vi "报表查询.vi"(11 "ConnectString":string="\"Provider=Microsoft.Jet.OLEDB.4.0;Data Source=C:\\\\Users\\\\Public\\\\Documents\\\\National \n\nInstruments\\\\TestStand 2017 (32-bit)\\\\Components\\\\Models\\\\TestStand Results.mdb;Persist Security Info=False\"") -> ()   [LabVIEW 2018, in "TestStand Simple UI.lvlib"]
uses:
  TestExec.llb/TestStand Simple UI.lvlib
  <vilib>/addons/database/Connection.llb/Conn ObjectReference.ctl
  <vilib>/addons/database/Connection.llb/DB Tools Open Connec (String).vi
  <vilib>/addons/database/Connection.llb/Conn Execute.vi
  <vilib>/addons/database/Recordset.llb/Rec Fetch Recordset Data (R).vi
  <vilib>/addons/database/Recordset.llb/Rec Destroy - Connection.vi
  <vilib>/Utility/file.llb/Write Delimited Spreadsheet (string).vi
  <vilib>/addons/database/_DB Variant To Data/Database Variant To Data.xnode
  <vilib>/addons/database/NI_Database_API.lvlib
panel:
  out "connection reference":T1
  out "error out":errorcluster
  in  "预览":bool
  in  "保存按钮":bool
  in  "搜索按钮":bool
  in  "二维码":string
  out "SN":string
  out "Row":i32
  in  "筛选结果":i32(listbox)
  in  "步骤结果":i32(listbox)
  in  "关键步骤":i32(listbox)
  out "data 2":string[][](array[string])
  out "tables":string[](array[string])
  in  "预览数据":i32(listbox)
  out "data 6":string[][](array[string])
  out "data 5":string[][](array[string])
  out "data 4":string[][](array[string])
  out "data 3":string[][](array[string])
  in  "测试报表":i32(listbox)
  out "data":string[][](array[string])
  in  "树形":string(tree)
  # "测试报表查询"
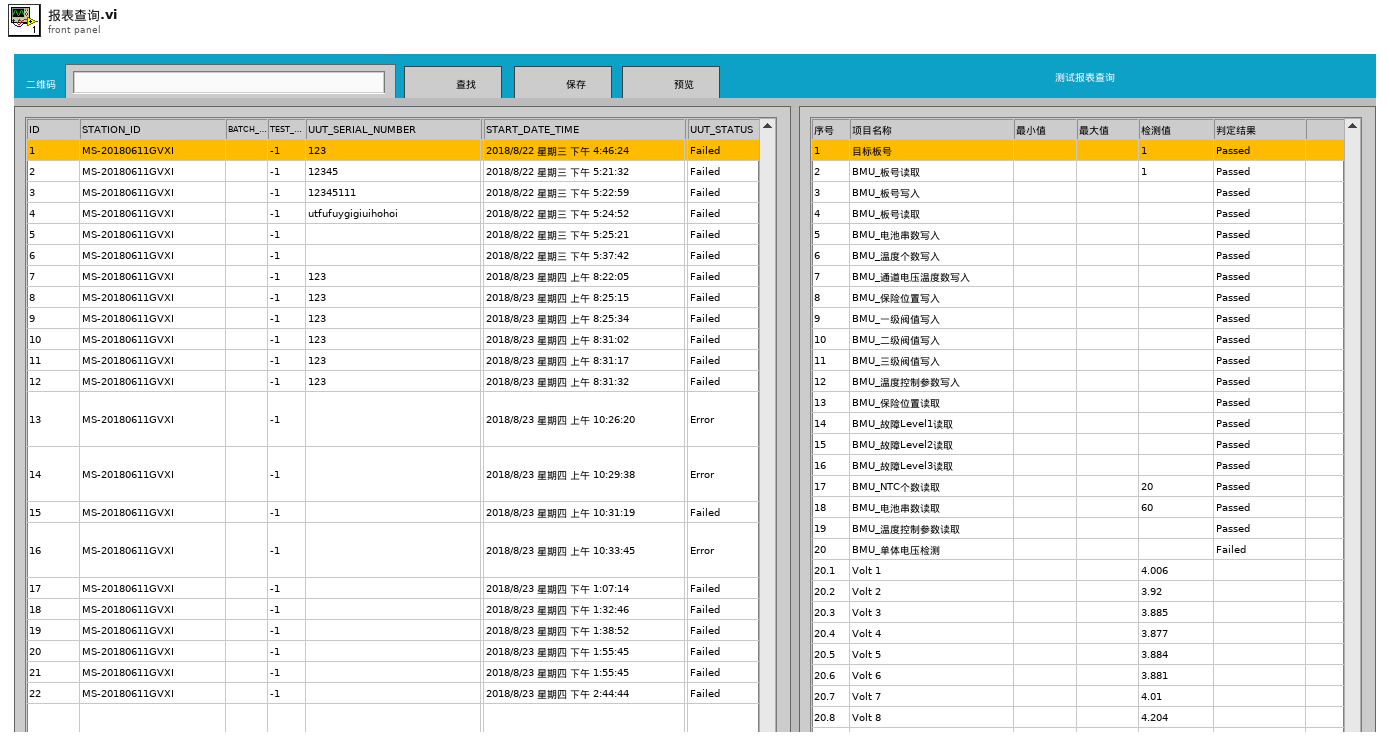
[diagram p1: front panel]
types:
  T1 = typedef "NI_Database_API.lvlib/Conn ObjectReference.ctl" = refnum<k1>
  T2 = typedef "LVPoint32TypeDef.ctl" = cluster{"Horizontal":i32, "Vertical":i32}
  T3 = typedef "LVRowAndColumnTypeDef.ctl" = cluster{"Row":i32, "Column":i32}
  T4 = typedef "NI_Database_API.lvlib/Rec ObjectReference.ctl" = refnum<k1>
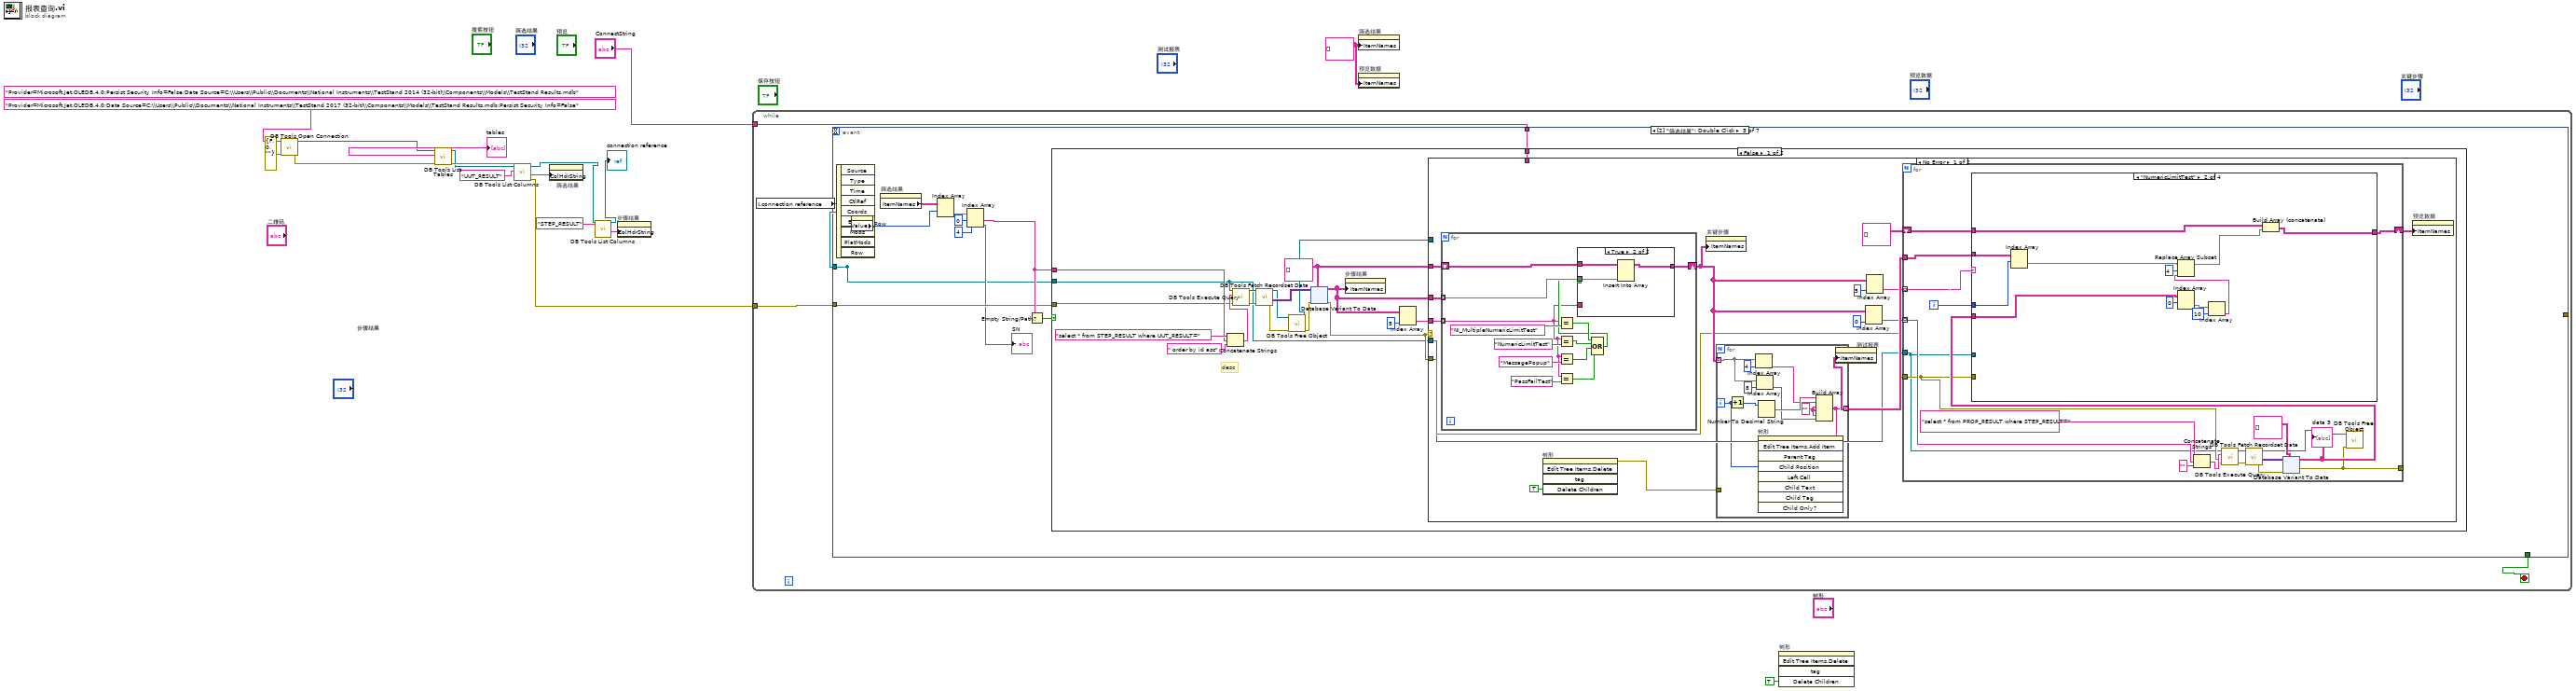
[diagram p0: block diagram]
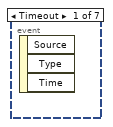
[diagram p2: hidden frame]
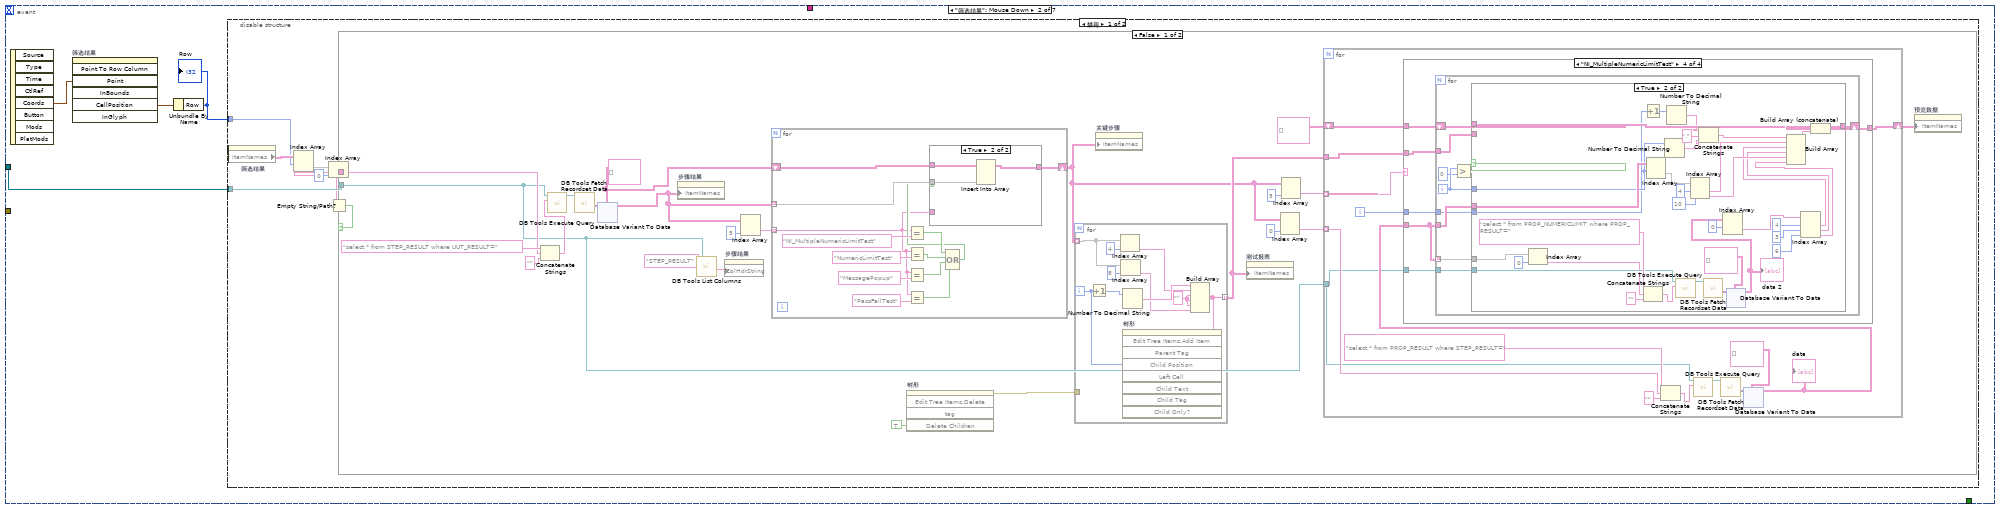
[diagram p3: hidden frame]
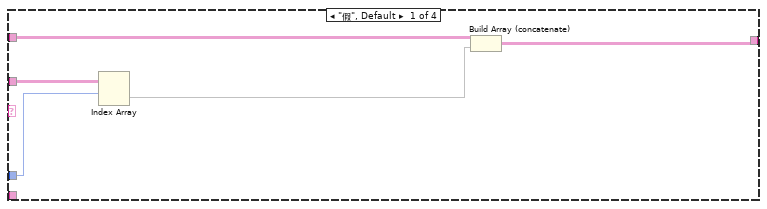
[diagram p4: hidden frame]
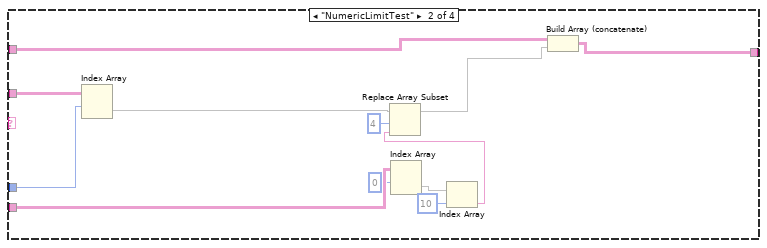
[diagram p5: hidden frame]
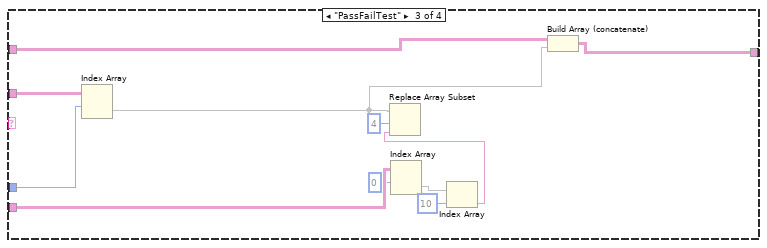
[diagram p6: hidden frame]
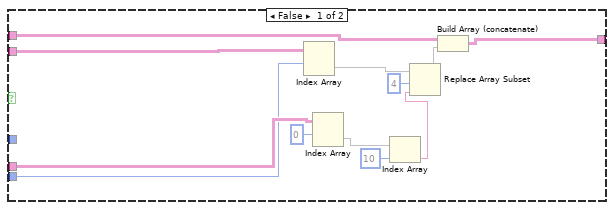
[diagram p7: hidden frame]
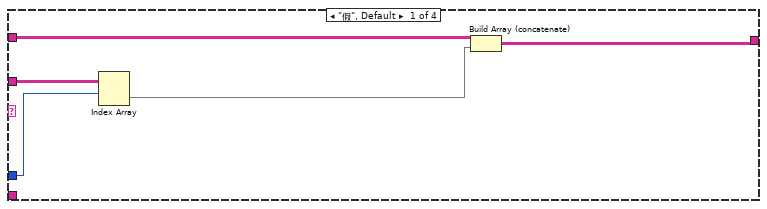
[diagram p11: hidden frame]
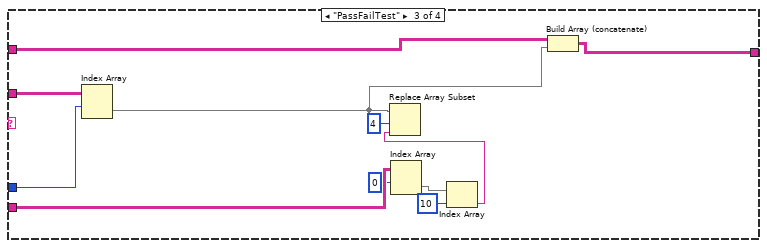
[diagram p12: hidden frame]
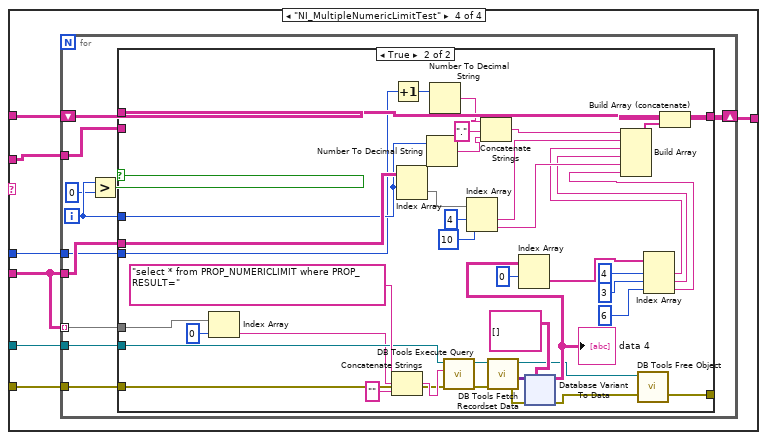
[diagram p13: hidden frame]
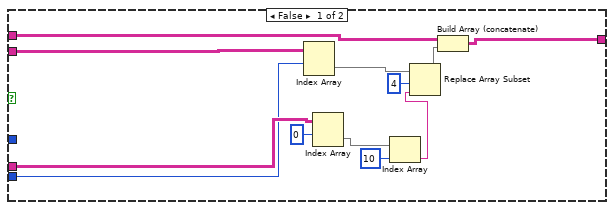
[diagram p14: hidden frame]
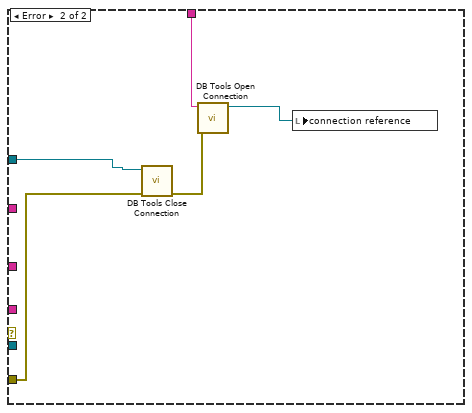
[diagram p16: hidden frame]
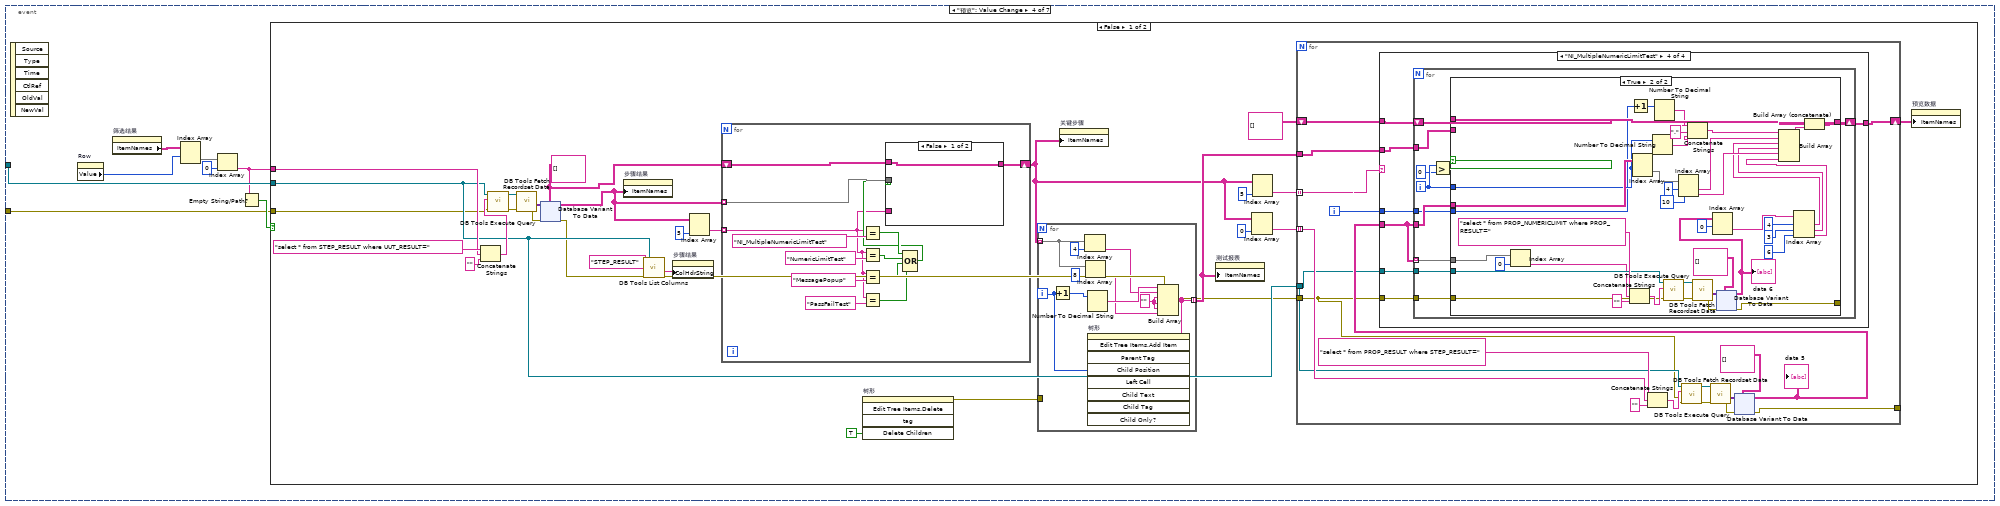
[diagram p18: hidden frame]
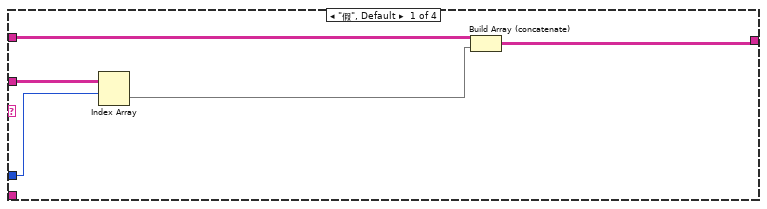
[diagram p19: hidden frame]
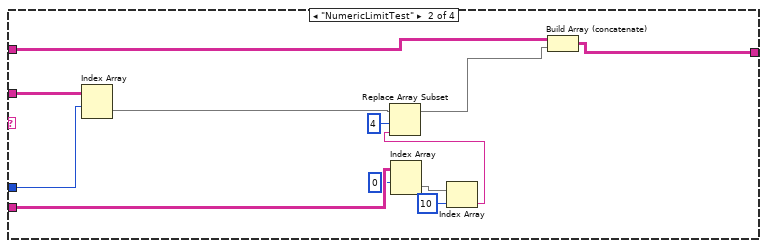
[diagram p20: hidden frame]
diagram:
  w2 = string[][] [] ("Item Names")
  (unwired) "Provider=Microsoft.Jet.OLEDB.4.0;Persist Security Info=False;Data Source=C:\\Users\\Public\\Documents\\National Instruments\\TestStand 2014 (32-bit)\\Components\\Models\\TestStand Results.mdb"
  n1 = call-poly <vilib>:"DB Tools Open Connection.vi"("error in (no error)"=errorcluster {"status"=FALSE, "code"=0, "source"=""}, "connection information"="Provider=Microsoft.Jet.OLEDB.4.0;Data Source=C:\\Users\\Public\\Documents\\National Instruments\\TestStand 2017 (32-bit)\\Components\\Models\\TestStand Results.mdb;Persist Security Info=False") -> ("error out"=w11:errorcluster, "connection reference"=w14:T1)  [unwired: 6 in]
  n2 = call <vilib>:"DB Tools List Tables.vi"("error in (no error)"=w11, "connection reference"=w14) -> ("error out"=w10:errorcluster, "tables"=→"tables":string[], "connection reference out"=w8:T1)  [unwired: 3 in]
  n3 = call <vilib>:"DB Tools List Columns.vi"("error in (no error)"=w10, "table"="UUT_RESULT", "connection reference"=w8) -> ("error out"=w9:errorcluster, "columns"=w15:string[], "connection reference out"=w5:T1)  [unwired: 1 in, 1 out]
  n4 = property on="筛选结果" class="MCListbox (strict)"("ColHdrString"=w15) -> ()  [unwired: 2 in, 2 out]
  n5 = call <vilib>:"DB Tools List Columns.vi"("table"="STEP_RESULT", "connection reference"=w5) -> ("columns"=w7:string[], "connection reference out"=→"connection reference":T1)  [unwired: 2 in, 2 out]
  n6 = property on="步骤结果" class="MCListbox (strict)"("ColHdrString"=w7) -> ()  [unwired: 2 in, 2 out]
  n7 = while {
    tunnel: w9 -> [w21]
    tunnel: "ConnectString" -> [w19]
    stop <- w20 stop-if-true
    n8 = local read "connection reference"() -> (w18:T1)
    n9 = event shown="[2] \"筛选结果\": Double Click" {
      selector: _ -> [_ _ _ _ _ _ _]
      dyn-events: _ -> [_ _ _ _ _ _ _]
      timeout: _ -> [_ _ _ _ _ _ _]
      tunnel: w18 -> [_ w23 w320 w650 _ w969 w974]
      tunnel: w21 -> [_ _ w324 w646 _ w968 w972]
      tunnel: [_ _ _ _ _ w970 _] -> w20
      tunnel: [_ _ _ _ _ _ w971] -> _
      tunnel: w19 -> [_ _ w321 _ _ _ _]
      tunnel: [_ _ w320 _ _ _ _] -> _
      event Timeout {
        n10 = event-data() -> ()  [unwired: 1 in, 3 out]
      }
      event "筛选结果": Mouse Down {
        n11 = event-data() -> ("Coords"=w25:T2)  [unwired: 1 in, 7 out]
        n12 = invoke on="筛选结果" class="MCListbox (严格)" method="Point To Row Column"("Point"=w25) -> ("CellPosition"=w24:T3)  [unwired: 6 in, 6 out]
        n13 = Unbundle By Name(w24) -> ("Row"=w22:i32)
        "Row" <- w22
        n14 = disable-structure shown="禁用" {
          disable-tunnel: w23 -> [w29 _]
          disable-tunnel: w22 -> [w28 _]
          frame Disabled {
            n15 = property on="筛选结果" class="MCListbox (strict)"() -> ("ItemNames"=w32:string[][])  [unwired: 2 in, 2 out]
            n16 = Index Array(array=w32, index (row)=w28) -> (element=w31:string[])  [unwired: 1 in]
            n17 = Index Array(array=w31, index=0 ("索引")) -> (element=w27:string)
            n18 = Empty String/Path?(string/path=w27) -> (empty?=w26:bool)
            n19 = case shown="False" w26 {
              tunnel: w29 -> [w37 _]
              tunnel: w27 -> [w49 _]
              frame False {
                w44 = string[][] []
                n20 = Concatenate Strings("select * from STEP_RESULT where UUT_RESULT=" ("condition"), w49, "" ("字符串")) -> (w51:string)
                n21 = call-poly <vilib>:"DB Tools Execute Query.vi"("SQL query"=w51, "connection reference"=w37) -> ("recordset reference"=w55:T4)  [unwired: 6 in, 1 out]
                n22 = call-poly <vilib>:"DB Tools Fetch Recordset Data.vi"("recordset reference"=w55) -> ("recordset data"=w54:variant[][])  [unwired: 4 in, 2 out]
                n23 = xnode "Database Variant To Data"("database variant"=w54, "type"=w44) -> ("data"=w45:string[][])  [unwired: 1 in, 1 out]
                n24 = property on="步骤结果" class="MCListbox (strict)"("ItemNames"=w45) -> ()  [unwired: 2 in, 2 out]
                n25 = call <vilib>:"DB Tools List Columns.vi"("table"="STEP_RESULT", "connection reference"=w37) -> ("columns"=w48:string[])  [unwired: 2 in, 3 out]
                n26 = property on="步骤结果" class="MCListbox (strict)"("ColHdrString"=w48) -> ()  [unwired: 2 in, 2 out]
                n27 = Index Array(array=w45, index (col)=5 ("禁用的索引 (列)")) -> (element=w46:string[])  [unwired: 1 in]
                n28 = for {
                  tunnel: w46 -> [w260] mode=indexing
                  tunnel: w45 -> [w264] mode=indexing
                  shift-right: [w262] -> w39
                  shift-left: w44 -> [w265]
                  n29 = Equal?(x=w260, y="NI_MultipleNumericLimitTest") -> (x = y?=w268:bool)
                  n30 = Equal?(x=w260, y="NumericLimitTest") -> (x = y?=w267:bool)
                  n31 = Equal?(x=w260, y="MessagePopup") -> (x = y?=w266:bool)
                  n32 = Equal?(x=w260, y="PassFailTest") -> (x = y?=w259:bool)
                  n33 = Compound Arithmetic op=OR(w268, w267, w266, w259) -> (w263:bool)
                  n34 = case shown="True" w263 {
                    tunnel: w265 -> [w272 w275]
                    tunnel: w264 -> [_ w274]
                    tunnel: [w272 w273] -> w262
                    tunnel: w260 -> [_ _]
                    frame False {
                    }
                    frame True {
                      n35 = Insert Into Array(array=w275, new element=w274) -> (w273:string[][])  [unwired: 2 in]
                    }
                  }
                }
                n36 = invoke on="树形" class="Tree (严格)" method="Edit Tree Items.Delete"("Delete Children"=TRUE ("删除子项？")) -> (error out=w35:errorcluster)  [unwired: 4 in, 4 out]
                n37 = for {
                  tunnel: w39 -> [w254] mode=indexing
                  tunnel: [w250] -> w43 mode=indexing
                  tunnel: w35 -> [_]
                  i -> [w249]
                  w252 = ""
                  n38 = Increment(x=w249) -> (x+1=w258:i32)
                  n39 = Index Array(array=w254, index=4 ("索引")) -> (element=w255:string)
                  n40 = Index Array(array=w254, index=8 ("索引")) -> (element=w251:string)
                  n41 = Number To Decimal String(number=w258) -> (decimal integer string=w257:string)  [unwired: 1 in]
                  n42 = Build Array(w257, w255, w252, w252, w252, w251) -> (w250:string[])
                  n43 = invoke on="树形" class="Tree (严格)" method="Edit Tree Items.Add Item"("Child Position"=w249, "Child Text"=w250) -> ()  [unwired: 7 in, 9 out]
                }
                n44 = property on="关键步骤" class="MCListbox (strict)"("ItemNames"=w39) -> ()  [unwired: 2 in, 2 out]
                n45 = property on="测试报表" class="MCListbox (strict)"("ItemNames"=w43) -> ()  [unwired: 2 in, 2 out]
                n46 = Index Array(array=w39, index (col)=0 ("禁用的索引 (列)")) -> (element=w38:string[])  [unwired: 1 in]
                n47 = Index Array(array=w39, index (col)=5 ("禁用的索引 (列)")) -> (element=w41:string[])  [unwired: 1 in]
                n48 = for {
                  tunnel: w41 -> [w69] mode=indexing
                  tunnel: w38 -> [w62] mode=indexing
                  tunnel: w37 -> [w56]
                  shift-right: [w58] -> w33
                  shift-left: string[][] [] -> [w59]
                  tunnel: w43 -> [w61]
                  i -> [w60]
                  n49 = Concatenate Strings("select * from PROP_RESULT where STEP_RESULT=" ("condition"), w62, "" ("字符串")) -> (w65:string)
                  n50 = call-poly <vilib>:"DB Tools Execute Query.vi"("SQL query"=w65, "connection reference"=w56) -> ("recordset reference"=w68:T4)  [unwired: 6 in, 1 out]
                  n51 = call-poly <vilib>:"DB Tools Fetch Recordset Data.vi"("recordset reference"=w68) -> ("recordset data"=w67:variant[][])  [unwired: 4 in, 2 out]
                  n52 = xnode "Database Variant To Data"("database variant"=w67, "type"=string[][] []) -> ("data"=w57:string[][])  [unwired: 1 in, 1 out]
                  "data" <- w57
                  n53 = case shown="\"NI_MultipleNumericLimitTest\"" w69 {
                    tunnel: w61 -> [w117 w123 w135 w143]
                    tunnel: w60 -> [w114 w122 w134 w147]
                    tunnel: w57 -> [_ w128 w140 w145]
                    tunnel: w59 -> [w118 w121 w133 w144]
                    tunnel: [w115 w119 w132 w146] -> w58
                    tunnel: w56 -> [_ _ _ w142]
                    frame "假", Default {
                      n54 = Index Array(array=w117, index (row)=w114) -> (element=w116:string[])  [unwired: 1 in]
                      n55 = Build Array (concatenate)(w118, w116) -> (w115:string[][])
                    }
                    frame "NumericLimitTest" {
                      n56 = Index Array(array=w123, index (row)=w122) -> (element=w130:string[])  [unwired: 1 in]
                      n57 = Index Array(array=w128, index (row)=0 ("索引 (行)")) -> (element=w126:string[])  [unwired: 1 in]
                      n58 = Index Array(array=w126, index=10 ("索引")) -> (element=w124:string)
                      n59 = Replace Array Subset(array=w130, new element=w124, index=4 ("索引")) -> (w120:string[])
                      n60 = Build Array (concatenate)(w121, w120) -> (w119:string[][])
                    }
                    frame "PassFailTest" {
                      n61 = Index Array(array=w135, index (row)=w134) -> (element=w131:string[])  [unwired: 1 in]
                      n62 = Index Array(array=w140, index (row)=0 ("索引 (行)")) -> (element=w138:string[])  [unwired: 1 in]
                      n63 = Index Array(array=w138, index=10 ("索引")) -> (element=w136:string)
                      n64 = Replace Array Subset(array=w131, new element=w136, index=4 ("索引")) -> ()  [unwired: 1 out]
                      n65 = Build Array (concatenate)(w133, w131) -> (w132:string[][])
                    }
                    frame "NI_MultipleNumericLimitTest" {
                      n66 = for {
                        tunnel: w145 -> [w157]
                        tunnel: w143 -> [w156]
                        tunnel: w147 -> [w155]
                        shift-right: [w153] -> w146
                        shift-left: w144 -> [w154]
                        tunnel: w145 -> [w148] mode=indexing
                        tunnel: w142 -> [w149]
                        i -> [w152]
                        n67 = Greater?(x=w152, y=0) -> (0:w151:bool)
                        n68 = case shown="True" w151 {
                          tunnel: w157 -> [w167 w201]
                          tunnel: w156 -> [w169 _]
                          tunnel: w155 -> [w166 w189]
                          tunnel: w154 -> [w160 w203]
                          tunnel: [w158 w202] -> w153
                          tunnel: w152 -> [_ w199]
                          tunnel: w149 -> [_ w182]
                          tunnel: w148 -> [_ w181]
                          frame False {
                            n69 = Index Array(array=w169, index (row)=w166) -> (element=w168:string[])  [unwired: 1 in]
                            n70 = Index Array(array=w167, index (row)=0 ("索引 (行)")) -> (element=w164:string[])  [unwired: 1 in]
                            n71 = Index Array(array=w164, index=10 ("索引")) -> (element=w161:string)
                            n72 = Replace Array Subset(array=w168, new element=w161, index=4 ("索引")) -> (w159:string[])
                            n73 = Build Array (concatenate)(w160, w159) -> (w158:string[][])
                          }
                          frame True {
                            n74 = Index Array(array=w181, index=0 ("索引")) -> (element=w179:string)
                            n75 = Concatenate Strings("select * from PROP_NUMERICLIMIT where PROP_RESULT=" ("condition"), w179, "" ("字符串")) -> (w186:string)
                            n76 = Increment(x=w189) -> (x+1=w190:i32)
                            n77 = Index Array(array=w201, index (row)=w199) -> (element=w200:string[])  [unwired: 1 in]
                            n78 = Number To Decimal String(number=w199) -> (decimal integer string=w192:string)  [unwired: 1 in]
                            n79 = Number To Decimal String(number=w190) -> (decimal integer string=w194:string)  [unwired: 1 in]
                            n80 = call-poly <vilib>:"DB Tools Execute Query.vi"("SQL query"=w186, "connection reference"=w182) -> ("recordset reference"=w183:T4)  [unwired: 6 in, 1 out]
                            n81 = Index Array(array=w200, index #1=4 ("索引"), index #2=10 ("索引")) -> (element #1=w197:string, element #2=w196:string)
                            n82 = Concatenate Strings(w194, "." ("字符串"), w192) -> (w191:string)
                            n83 = call-poly <vilib>:"DB Tools Fetch Recordset Data.vi"("recordset reference"=w183) -> ("recordset data"=w184:variant[][])  [unwired: 4 in, 2 out]
                            n84 = xnode "Database Variant To Data"("database variant"=w184, "type"=string[][] []) -> ("data"=w177:string[][])  [unwired: 1 in, 1 out]
                            "data 2" <- w177
                            n85 = Index Array(array=w177, index (row)=0 ("索引")) -> (element=w176:string[])  [unwired: 1 in]
                            n86 = Index Array(array=w176, index #1=4 ("索引"), index #2=3 ("索引"), index #3=6 ("索引")) -> (element #1=w172:string, element #2=w171:string, element #3=w170:string)
                            n87 = Build Array(w191, w197, w172, w171, w196, w170) -> (w195:string[])
                            n88 = Build Array (concatenate)(w203, w195) -> (w202:string[][])
                          }
                        }
                      }
                    }
                  }
                }
                n89 = property on="预览数据" class="MCListbox (strict)"("ItemNames"=w33) -> ()  [unwired: 2 in, 2 out]
              }
              frame True {
              }
            }
          }
          frame Enabled {
          }
        }
      }
      event "筛选结果": Double Click {
        n90 = event-data() -> ()  [unwired: 1 in, 9 out]
        n91 = property on="Row" class="DigNum (strict)"() -> ("Value"=w325:i32)  [unwired: 2 in, 2 out]
        n92 = property on="筛选结果" class="MCListbox (strict)"() -> ("ItemNames"=w330:string[][])  [unwired: 2 in, 2 out]
        n93 = Index Array(array=w330, index (row)=w325) -> (element=w329:string[])  [unwired: 1 in]
        n94 = Index Array(array=w329, index #1=0 ("索引"), index #2=4 ("索引")) -> (element #1=w327:string, element #2=→"SN":string)
        n95 = Empty String/Path?(string/path=w327) -> (empty?=w326:bool)
        n96 = case shown="False" w326 {
          tunnel: w320 -> [w335 _]
          tunnel: w327 -> [w344 _]
          tunnel: w324 -> [w336 _]
          tunnel: w321 -> [w338 _]
          frame False {
            w340 = string[][] []
            # "desc"
            n97 = Concatenate Strings("select * from STEP_RESULT where UUT_RESULT=" ("condition"), w344, " order by id asc" ("字符串")) -> (w345:string)
            n98 = call-poly <vilib>:"DB Tools Execute Query.vi"("error in (no error)"=w336, "SQL query"=w345, "connection reference"=w335) -> ("error out"=w339:errorcluster, "recordset reference"=w349:T4)  [unwired: 5 in]
            n99 = call-poly <vilib>:"DB Tools Fetch Recordset Data.vi"("error in (no error)"=w339, "recordset reference"=w349) -> ("error out"=w333:errorcluster, "recordset data"=w348:variant[][], "recordset reference out"=w334:T4)  [unwired: 3 in]
            n100 = call-poly <vilib>:"DB Tools Free Object.vi"("error in (no error)"=w333, "recordset reference"=w334) -> ("error out"=w332:errorcluster, "connection reference"=w331:T1)  [unwired: 8 in]
            n101 = xnode "Database Variant To Data"("database variant"=w348, "error in (no error)"=w332, "type"=w340) -> ("data"=w341:string[][], "error out"=w337:errorcluster)
            n102 = property on="步骤结果" class="MCListbox (strict)"("ItemNames"=w341) -> ()  [unwired: 2 in, 2 out]
            n103 = Index Array(array=w341, index (col)=5 ("禁用的索引 (列)")) -> (element=w342:string[])  [unwired: 1 in]
            n104 = case shown="No Error" w337 {
              tunnel: w342 -> [w364 _]
              tunnel: w341 -> [w363 _]
              tunnel: w340 -> [w362 _]
              tunnel: w337 -> [w351 w597]
              tunnel: w338 -> [_ w601]
              tunnel: w335 -> [w350 _]
              tunnel: w331 -> [_ w598]
              frame No Error {
                n105 = for {
                  tunnel: w364 -> [w581] mode=indexing
                  tunnel: w363 -> [w585] mode=indexing
                  shift-right: [w583] -> w357
                  shift-left: w362 -> [w586]
                  n106 = Equal?(x=w581, y="NI_MultipleNumericLimitTest") -> (x = y?=w589:bool)
                  n107 = Equal?(x=w581, y="NumericLimitTest") -> (x = y?=w588:bool)
                  n108 = Equal?(x=w581, y="MessagePopup") -> (x = y?=w587:bool)
                  n109 = Equal?(x=w581, y="PassFailTest") -> (x = y?=w580:bool)
                  n110 = Compound Arithmetic op=OR(w589, w588, w587, w580) -> (w584:bool)
                  n111 = case shown="True" w584 {
                    tunnel: w586 -> [w593 w596]
                    tunnel: w585 -> [_ w595]
                    tunnel: [w593 w594] -> w583
                    tunnel: w581 -> [_ _]
                    frame False {
                    }
                    frame True {
                      n112 = Insert Into Array(array=w596, new element=w595) -> (w594:string[][])  [unwired: 2 in]
                    }
                  }
                }
                n113 = invoke on="树形" class="Tree (严格)" method="Edit Tree Items.Delete"("Delete Children"=TRUE ("删除子项？")) -> (error out=w354:errorcluster)  [unwired: 4 in, 4 out]
                n114 = property on="关键步骤" class="MCListbox (strict)"("ItemNames"=w357) -> ()  [unwired: 2 in, 2 out]
                n115 = for {
                  tunnel: w357 -> [w575] mode=indexing
                  tunnel: [w571] -> w361 mode=indexing
                  tunnel: w354 -> [_]
                  i -> [w570]
                  w573 = ""
                  n116 = Increment(x=w570) -> (x+1=w579:i32)
                  n117 = Index Array(array=w575, index=4 ("索引")) -> (element=w576:string)
                  n118 = Index Array(array=w575, index=8 ("索引")) -> (element=w572:string)
                  n119 = Number To Decimal String(number=w579) -> (decimal integer string=w578:string)  [unwired: 1 in]
                  n120 = Build Array(w578, w576, w573, w573, w573, w572) -> (w571:string[])
                  n121 = invoke on="树形" class="Tree (严格)" method="Edit Tree Items.Add Item"("Child Position"=w570, "Child Text"=w571) -> ()  [unwired: 7 in, 9 out]
                }
                n122 = property on="测试报表" class="MCListbox (strict)"("ItemNames"=w361) -> ()  [unwired: 2 in, 2 out]
                n123 = Index Array(array=w357, index (col)=0 ("禁用的索引 (列)")) -> (element=w356:string[])  [unwired: 1 in]
                n124 = Index Array(array=w357, index (col)=5 ("禁用的索引 (列)")) -> (element=w359:string[])  [unwired: 1 in]
                n125 = for {
                  tunnel: w359 -> [w383] mode=indexing
                  tunnel: w356 -> [w376] mode=indexing
                  tunnel: w350 -> [w365]
                  shift-right: [w372] -> w352
                  shift-left: string[][] [] -> [w373]
                  tunnel: w361 -> [w375]
                  tunnel: w351 -> [w370]
                  tunnel: [w366] -> _
                  i -> [w374]
                  n126 = Concatenate Strings("select * from PROP_RESULT where STEP_RESULT=" ("condition"), w376, "" ("字符串")) -> (w379:string)
                  n127 = call-poly <vilib>:"DB Tools Execute Query.vi"("error in (no error)"=w370, "SQL query"=w379, "connection reference"=w365) -> ("error out"=w369:errorcluster, "recordset reference"=w382:T4)  [unwired: 5 in]
                  n128 = call-poly <vilib>:"DB Tools Fetch Recordset Data.vi"("error in (no error)"=w369, "recordset reference"=w382) -> ("error out"=w368:errorcluster, "recordset data"=w381:variant[][], "recordset reference out"=w367:T4)  [unwired: 3 in]
                  n129 = xnode "Database Variant To Data"("database variant"=w381, "error in (no error)"=w368, "type"=string[][] []) -> ("data"=w371:string[][], "error out"=w366:errorcluster)
                  "data 3" <- w371
                  n130 = case shown="\"NumericLimitTest\"" w383 {
                    tunnel: w375 -> [w431 w437 w449 w458]
                    tunnel: w374 -> [w428 w436 w448 w462]
                    tunnel: w371 -> [_ w442 w454 w460]
                    tunnel: w373 -> [w432 w435 w447 w459]
                    tunnel: [w429 w433 w446 w461] -> w372
                    tunnel: w365 -> [_ _ _ w457]
                    tunnel: w370 -> [_ _ _ w456]
                    frame "假", Default {
                      n131 = Index Array(array=w431, index (row)=w428) -> (element=w430:string[])  [unwired: 1 in]
                      n132 = Build Array (concatenate)(w432, w430) -> (w429:string[][])
                    }
                    frame "NumericLimitTest" {
                      n133 = Index Array(array=w437, index (row)=w436) -> (element=w444:string[])  [unwired: 1 in]
                      n134 = Index Array(array=w442, index (row)=0 ("索引 (行)")) -> (element=w440:string[])  [unwired: 1 in]
                      n135 = Index Array(array=w440, index=10 ("索引")) -> (element=w438:string)
                      n136 = Replace Array Subset(array=w444, new element=w438, index=4 ("索引")) -> (w434:string[])
                      n137 = Build Array (concatenate)(w435, w434) -> (w433:string[][])
                    }
                    frame "PassFailTest" {
                      n138 = Index Array(array=w449, index (row)=w448) -> (element=w445:string[])  [unwired: 1 in]
                      n139 = Index Array(array=w454, index (row)=0 ("索引 (行)")) -> (element=w452:string[])  [unwired: 1 in]
                      n140 = Index Array(array=w452, index=10 ("索引")) -> (element=w450:string)
                      n141 = Replace Array Subset(array=w445, new element=w450, index=4 ("索引")) -> ()  [unwired: 1 out]
                      n142 = Build Array (concatenate)(w447, w445) -> (w446:string[][])
                    }
                    frame "NI_MultipleNumericLimitTest" {
                      n143 = for {
                        tunnel: w460 -> [w473]
                        tunnel: w458 -> [w472]
                        tunnel: w462 -> [w471]
                        shift-right: [w469] -> w461
                        shift-left: w459 -> [w470]
                        tunnel: w460 -> [w464] mode=indexing
                        tunnel: w457 -> [w465]
                        tunnel: w456 -> [w463]
                        i -> [w468]
                        n144 = Greater?(x=w468, y=0) -> (0:w467:bool)
                        n145 = case shown="True" w467 {
                          tunnel: w473 -> [w483 w522]
                          tunnel: w472 -> [w485 _]
                          tunnel: w471 -> [w482 w510]
                          tunnel: w470 -> [w476 w524]
                          tunnel: [w474 w523] -> w469
                          tunnel: w468 -> [_ w520]
                          tunnel: w465 -> [_ w503]
                          tunnel: w464 -> [_ w502]
                          tunnel: w463 -> [_ w490]
                          tunnel: [_ w487] -> _
                          frame False {
                            n146 = Index Array(array=w485, index (row)=w482) -> (element=w484:string[])  [unwired: 1 in]
                            n147 = Index Array(array=w483, index (row)=0 ("索引 (行)")) -> (element=w480:string[])  [unwired: 1 in]
                            n148 = Index Array(array=w480, index=10 ("索引")) -> (element=w477:string)
                            n149 = Replace Array Subset(array=w484, new element=w477, index=4 ("索引")) -> (w475:string[])
                            n150 = Build Array (concatenate)(w476, w475) -> (w474:string[][])
                          }
                          frame True {
                            n151 = Index Array(array=w502, index=0 ("索引")) -> (element=w500:string)
                            n152 = Concatenate Strings("select * from PROP_NUMERICLIMIT where PROP_RESULT=" ("condition"), w500, "" ("字符串")) -> (w507:string)
                            n153 = Increment(x=w510) -> (x+1=w511:i32)
                            n154 = Index Array(array=w522, index (row)=w520) -> (element=w521:string[])  [unwired: 1 in]
                            n155 = Number To Decimal String(number=w520) -> (decimal integer string=w513:string)  [unwired: 1 in]
                            n156 = Number To Decimal String(number=w511) -> (decimal integer string=w515:string)  [unwired: 1 in]
                            n157 = call-poly <vilib>:"DB Tools Execute Query.vi"("error in (no error)"=w490, "SQL query"=w507, "connection reference"=w503) -> ("error out"=w489:errorcluster, "recordset reference"=w504:T4)  [unwired: 5 in]
                            n158 = Index Array(array=w521, index #1=4 ("索引"), index #2=10 ("索引")) -> (element #1=w518:string, element #2=w517:string)
                            n159 = Concatenate Strings(w515, "." ("字符串"), w513) -> (w512:string)
                            n160 = call-poly <vilib>:"DB Tools Fetch Recordset Data.vi"("error in (no error)"=w489, "recordset reference"=w504) -> ("error out"=w488:errorcluster, "recordset data"=w505:variant[][], "recordset reference out"=w486:T4)  [unwired: 3 in]
                            n161 = xnode "Database Variant To Data"("database variant"=w505, "error in (no error)"=w488, "type"=string[][] []) -> ("data"=w498:string[][], "error out"=w487:errorcluster)
                            "data 4" <- w498
                            n162 = Index Array(array=w498, index (row)=0 ("索引")) -> (element=w497:string[])  [unwired: 1 in]
                            n163 = call-poly <vilib>:"DB Tools Free Object.vi"("recordset reference"=w486) -> ()  [unwired: 9 in, 2 out]
                            n164 = Index Array(array=w497, index #1=4 ("索引"), index #2=3 ("索引"), index #3=6 ("索引")) -> (element #1=w493:string, element #2=w492:string, element #3=w491:string)
                            n165 = Build Array(w512, w518, w493, w492, w517, w491) -> (w516:string[])
                            n166 = Build Array (concatenate)(w524, w516) -> (w523:string[][])
                          }
                        }
                      }
                    }
                  }
                  n167 = call-poly <vilib>:"DB Tools Free Object.vi"("error in (no error)"=w366, "recordset reference"=w367) -> ()  [unwired: 8 in, 2 out]
                }
                n168 = property on="预览数据" class="MCListbox (strict)"("ItemNames"=w352) -> ()  [unwired: 2 in, 2 out]
              }
              frame Error {
                n169 = call <vilib>:"DB Tools Close Connection.vi"("error in (no error)"=w597, "connection reference"=w598) -> ("error out"=w599:errorcluster)  [unwired: 5 in]
                n170 = call-poly <vilib>:"DB Tools Open Connection.vi"("error in (no error)"=w599, "connection information"=w601) -> ("connection reference"=w600:T1)  [unwired: 6 in, 1 out]
                n171 = local write "connection reference"(w600) -> ()
              }
            }
          }
          frame True {
          }
        }
      }
      event "预览": Value Change {
        n172 = event-data() -> ()  [unwired: 1 in, 6 out]
        n173 = property on="Row" class="DigNum (strict)"() -> ("Value"=w647:i32)  [unwired: 2 in, 2 out]
        n174 = property on="筛选结果" class="MCListbox (strict)"() -> ("ItemNames"=w653:string[][])  [unwired: 2 in, 2 out]
        n175 = Index Array(array=w653, index (row)=w647) -> (element=w652:string[])  [unwired: 1 in]
        n176 = Index Array(array=w652, index=0 ("索引")) -> (element=w649:string)
        n177 = Empty String/Path?(string/path=w649) -> (empty?=w648:bool)
        n178 = case shown="False" w648 {
          tunnel: w650 -> [w663 _]
          tunnel: w649 -> [w675 _]
          tunnel: w646 -> [w658 _]
          frame False {
            w670 = string[][] []
            n179 = Concatenate Strings("select * from STEP_RESULT where UUT_RESULT=" ("condition"), w675, "" ("字符串")) -> (w677:string)
            n180 = call-poly <vilib>:"DB Tools Execute Query.vi"("error in (no error)"=w658, "SQL query"=w677, "connection reference"=w663) -> ("error out"=w657:errorcluster, "recordset reference"=w681:T4)  [unwired: 5 in]
            n181 = call-poly <vilib>:"DB Tools Fetch Recordset Data.vi"("error in (no error)"=w657, "recordset reference"=w681) -> ("error out"=w656:errorcluster, "recordset data"=w680:variant[][])  [unwired: 3 in, 1 out]
            n182 = xnode "Database Variant To Data"("database variant"=w680, "error in (no error)"=w656, "type"=w670) -> ("data"=w671:string[][], "error out"=w655:errorcluster)
            n183 = property on="步骤结果" class="MCListbox (strict)"("ItemNames"=w671) -> ()  [unwired: 2 in, 2 out]
            n184 = call <vilib>:"DB Tools List Columns.vi"("error in (no error)"=w655, "table"="STEP_RESULT", "connection reference"=w663) -> ("error out"=w654:errorcluster, "columns"=w674:string[])  [unwired: 1 in, 2 out]
            n185 = property on="步骤结果" class="MCListbox (strict)"("ColHdrString"=w674) -> ()  [unwired: 2 in, 2 out]
            n186 = Index Array(array=w671, index (col)=5 ("禁用的索引 (列)")) -> (element=w672:string[])  [unwired: 1 in]
            n187 = for {
              tunnel: w672 -> [w896] mode=indexing
              tunnel: w671 -> [w900] mode=indexing
              shift-right: [w898] -> w665
              shift-left: w670 -> [w901]
              n188 = Equal?(x=w896, y="NI_MultipleNumericLimitTest") -> (x = y?=w904:bool)
              n189 = Equal?(x=w896, y="NumericLimitTest") -> (x = y?=w903:bool)
              n190 = Equal?(x=w896, y="MessagePopup") -> (x = y?=w902:bool)
              n191 = Equal?(x=w896, y="PassFailTest") -> (x = y?=w895:bool)
              n192 = Compound Arithmetic op=OR(w904, w903, w902, w895) -> (w899:bool)
              n193 = case shown="False" w899 {
                tunnel: w901 -> [w908 w911]
                tunnel: w900 -> [_ w910]
                tunnel: [w908 w909] -> w898
                tunnel: w896 -> [_ _]
                frame False {
                }
                frame True {
                  n194 = Insert Into Array(array=w911, new element=w910) -> (w909:string[][])  [unwired: 2 in]
                }
              }
            }
            n195 = invoke on="树形" class="Tree (严格)" method="Edit Tree Items.Delete"("Delete Children"=TRUE ("删除子项？")) -> (error out=w661:errorcluster)  [unwired: 4 in, 4 out]
            n196 = for {
              tunnel: w665 -> [w890] mode=indexing
              tunnel: [w886] -> w669 mode=indexing
              tunnel: w661 -> [_]
              i -> [w885]
              w888 = ""
              n197 = Increment(x=w885) -> (x+1=w894:i32)
              n198 = Index Array(array=w890, index=4 ("索引")) -> (element=w891:string)
              n199 = Index Array(array=w890, index=8 ("索引")) -> (element=w887:string)
              n200 = Number To Decimal String(number=w894) -> (decimal integer string=w893:string)  [unwired: 1 in]
              n201 = Build Array(w893, w891, w888, w888, w888, w887) -> (w886:string[])
              n202 = invoke on="树形" class="Tree (严格)" method="Edit Tree Items.Add Item"("Child Position"=w885, "Child Text"=w886) -> ()  [unwired: 7 in, 9 out]
            }
            n203 = property on="关键步骤" class="MCListbox (strict)"("ItemNames"=w665) -> ()  [unwired: 2 in, 2 out]
            n204 = property on="测试报表" class="MCListbox (strict)"("ItemNames"=w669) -> ()  [unwired: 2 in, 2 out]
            n205 = Index Array(array=w665, index (col)=0 ("禁用的索引 (列)")) -> (element=w664:string[])  [unwired: 1 in]
            n206 = Index Array(array=w665, index (col)=5 ("禁用的索引 (列)")) -> (element=w667:string[])  [unwired: 1 in]
            n207 = for {
              tunnel: w667 -> [w699] mode=indexing
              tunnel: w664 -> [w692] mode=indexing
              tunnel: w663 -> [w686]
              shift-right: [w688] -> w659
              shift-left: string[][] [] -> [w689]
              tunnel: w669 -> [w691]
              tunnel: w654 -> [w685]
              tunnel: [w682] -> _
              i -> [w690]
              n208 = Concatenate Strings("select * from PROP_RESULT where STEP_RESULT=" ("condition"), w692, "" ("字符串")) -> (w695:string)
              n209 = call-poly <vilib>:"DB Tools Execute Query.vi"("error in (no error)"=w685, "SQL query"=w695, "connection reference"=w686) -> ("error out"=w684:errorcluster, "recordset reference"=w698:T4)  [unwired: 5 in]
              n210 = call-poly <vilib>:"DB Tools Fetch Recordset Data.vi"("error in (no error)"=w684, "recordset reference"=w698) -> ("error out"=w683:errorcluster, "recordset data"=w697:variant[][])  [unwired: 3 in, 1 out]
              n211 = xnode "Database Variant To Data"("database variant"=w697, "error in (no error)"=w683, "type"=string[][] []) -> ("data"=w687:string[][], "error out"=w682:errorcluster)
              "data 5" <- w687
              n212 = case shown="\"NI_MultipleNumericLimitTest\"" w699 {
                tunnel: w691 -> [w747 w753 w765 w774]
                tunnel: w690 -> [w744 w752 w764 w778]
                tunnel: w687 -> [_ w758 w770 w776]
                tunnel: w689 -> [w748 w751 w763 w775]
                tunnel: [w745 w749 w762 w777] -> w688
                tunnel: w686 -> [_ _ _ w773]
                tunnel: w685 -> [_ _ _ w772]
                frame "假", Default {
                  n213 = Index Array(array=w747, index (row)=w744) -> (element=w746:string[])  [unwired: 1 in]
                  n214 = Build Array (concatenate)(w748, w746) -> (w745:string[][])
                }
                frame "NumericLimitTest" {
                  n215 = Index Array(array=w753, index (row)=w752) -> (element=w760:string[])  [unwired: 1 in]
                  n216 = Index Array(array=w758, index (row)=0 ("索引 (行)")) -> (element=w756:string[])  [unwired: 1 in]
                  n217 = Index Array(array=w756, index=10 ("索引")) -> (element=w754:string)
                  n218 = Replace Array Subset(array=w760, new element=w754, index=4 ("索引")) -> (w750:string[])
                  n219 = Build Array (concatenate)(w751, w750) -> (w749:string[][])
                }
                frame "PassFailTest" {
                  n220 = Index Array(array=w765, index (row)=w764) -> (element=w761:string[])  [unwired: 1 in]
                  n221 = Index Array(array=w770, index (row)=0 ("索引 (行)")) -> (element=w768:string[])  [unwired: 1 in]
                  n222 = Index Array(array=w768, index=10 ("索引")) -> (element=w766:string)
                  n223 = Replace Array Subset(array=w761, new element=w766, index=4 ("索引")) -> ()  [unwired: 1 out]
                  n224 = Build Array (concatenate)(w763, w761) -> (w762:string[][])
                }
                frame "NI_MultipleNumericLimitTest" {
                  n225 = for {
                    tunnel: w776 -> [w789]
                    tunnel: w774 -> [w788]
                    tunnel: w778 -> [w787]
                    shift-right: [w785] -> w777
                    shift-left: w775 -> [w786]
                    tunnel: w776 -> [w780] mode=indexing
                    tunnel: w773 -> [w781]
                    tunnel: w772 -> [w779]
                    i -> [w784]
                    n226 = Greater?(x=w784, y=0) -> (0:w783:bool)
                    n227 = case shown="True" w783 {
                      tunnel: w789 -> [w799 w837]
                      tunnel: w788 -> [w801 _]
                      tunnel: w787 -> [w798 w825]
                      tunnel: w786 -> [w792 w839]
                      tunnel: [w790 w838] -> w785
                      tunnel: w784 -> [_ w835]
                      tunnel: w781 -> [_ w818]
                      tunnel: w780 -> [_ w817]
                      tunnel: w779 -> [_ w805]
                      tunnel: [_ w802] -> _
                      frame False {
                        n228 = Index Array(array=w801, index (row)=w798) -> (element=w800:string[])  [unwired: 1 in]
                        n229 = Index Array(array=w799, index (row)=0 ("索引 (行)")) -> (element=w796:string[])  [unwired: 1 in]
                        n230 = Index Array(array=w796, index=10 ("索引")) -> (element=w793:string)
                        n231 = Replace Array Subset(array=w800, new element=w793, index=4 ("索引")) -> (w791:string[])
                        n232 = Build Array (concatenate)(w792, w791) -> (w790:string[][])
                      }
                      frame True {
                        n233 = Index Array(array=w817, index=0 ("索引")) -> (element=w815:string)
                        n234 = Concatenate Strings("select * from PROP_NUMERICLIMIT where PROP_RESULT=" ("condition"), w815, "" ("字符串")) -> (w822:string)
                        n235 = Increment(x=w825) -> (x+1=w826:i32)
                        n236 = Index Array(array=w837, index (row)=w835) -> (element=w836:string[])  [unwired: 1 in]
                        n237 = Number To Decimal String(number=w835) -> (decimal integer string=w828:string)  [unwired: 1 in]
                        n238 = Number To Decimal String(number=w826) -> (decimal integer string=w830:string)  [unwired: 1 in]
                        n239 = call-poly <vilib>:"DB Tools Execute Query.vi"("error in (no error)"=w805, "SQL query"=w822, "connection reference"=w818) -> ("error out"=w804:errorcluster, "recordset reference"=w819:T4)  [unwired: 5 in]
                        n240 = Index Array(array=w836, index #1=4 ("索引"), index #2=10 ("索引")) -> (element #1=w833:string, element #2=w832:string)
                        n241 = Concatenate Strings(w830, "." ("字符串"), w828) -> (w827:string)
                        n242 = call-poly <vilib>:"DB Tools Fetch Recordset Data.vi"("error in (no error)"=w804, "recordset reference"=w819) -> ("error out"=w803:errorcluster, "recordset data"=w820:variant[][])  [unwired: 3 in, 1 out]
                        n243 = xnode "Database Variant To Data"("database variant"=w820, "error in (no error)"=w803, "type"=string[][] []) -> ("data"=w813:string[][], "error out"=w802:errorcluster)
                        "data 6" <- w813
                        n244 = Index Array(array=w813, index (row)=0 ("索引")) -> (element=w812:string[])  [unwired: 1 in]
                        n245 = Index Array(array=w812, index #1=4 ("索引"), index #2=3 ("索引"), index #3=6 ("索引")) -> (element #1=w808:string, element #2=w807:string, element #3=w806:string)
                        n246 = Build Array(w827, w833, w808, w807, w832, w806) -> (w831:string[])
                        n247 = Build Array (concatenate)(w839, w831) -> (w838:string[][])
                      }
                    }
                  }
                }
              }
            }
            n248 = property on="预览数据" class="MCListbox (strict)"("ItemNames"=w659) -> ()  [unwired: 2 in, 2 out]
          }
          frame True {
          }
        }
      }
      event "保存按钮": Value Change {
        n249 = event-data() -> ("NewVal"=w956:bool)  [unwired: 1 in, 5 out]
        n250 = case shown="True" w956 {
          frame False {
          }
          frame True {
            w958 = "*.csv" ("pattern (all files)")
            n251 = property on="SN" class="Str"() -> ("Value"=w959:string)  [unwired: 2 in, 2 out]
            n252 = call "文件对话框"("start path"=path "D:/", "default name"=w959, "pattern (all files)"=w958, "pattern label"=w958) -> ("selected path"=w960:path)  [unwired: 8 in, 3 out]
            n253 = Not A Number/Path/Refnum?(number/path/refnum=w960) -> (NaN/Path/Refnum?=w961:bool)
            n254 = case shown="False" w961 {
              tunnel: w960 -> [w964 _]
              frame False {
                n255 = property on="预览数据" class="MCListbox (strict)"() -> ("ItemNames"=w965:string[][])  [unwired: 2 in, 2 out]
                n256 = property on="预览数据" class="MCListbox (strict)"() -> ("ColHdrString"=w966:string[])  [unwired: 2 in, 2 out]
                n257 = Build Array (concatenate)(w966, w965) -> (w962:string[][])
                n258 = call-poly <vilib>:"Write Delimited Spreadsheet.vi"("file path (dialog if empty)"=w964, "2D data"=w962, "delimiter (\\t)"="," ("delimiter (\\t)")) -> ()  [unwired: 11 in, 2 out]
              }
              frame True {
              }
            }
          }
        }
      }
      event Panel Close? {
        w970 = TRUE ("Discard?")
        n259 = event-data() -> ()  [unwired: 1 in, 4 out]
        n260 = call <vilib>:"DB Tools Close Connection.vi"("error in (no error)"=w968, "connection reference"=w969) -> ("error out"=→"error out":errorcluster)  [unwired: 5 in]
        n261 = event-data("Discard?"=w970) -> ()  [unwired: 1 in, 1 out]
      }
      event "搜索按钮": Value Change {
        n262 = event-data() -> ("NewVal"=w973:bool)  [unwired: 1 in, 5 out]
        n263 = case shown="False" w973 {
          tunnel: w974 -> [_ w980]
          tunnel: w972 -> [w975 w978]
          tunnel: [w975 w976] -> w971
          frame False {
          }
          frame True {
            n264 = property on="二维码" class="Str"() -> ("Value"=w992:string)  [unwired: 2 in, 2 out]
            n265 = call <vilib>:"Trim Whitespace.vi"("string"=w992) -> ("trimmed string"=w988:string)  [unwired: 1 in]
            n266 = Empty String/Path?(string/path=w988) -> (empty?=w984:bool)
            n267 = Concatenate Strings("select * from UUT_RESULT where UUT_SERIAL_NUMBER=\"" ("condition"), w988, "\"" ("字符串")) -> (w990:string)
            n268 = Select(t="select * from UUT_RESULT" ("condition"), s=w984, f=w990) -> (s? t:f=w986:string)
            n269 = call-poly <vilib>:"DB Tools Execute Query.vi"("error in (no error)"=w978, "SQL query"=w986, "connection reference"=w980) -> ("error out"=w979:errorcluster, "recordset reference"=w991:T4)  [unwired: 5 in]
            n270 = call-poly <vilib>:"DB Tools Fetch Recordset Data.vi"("error in (no error)"=w979, "recordset reference"=w991) -> ("error out"=w977:errorcluster, "recordset data"=w983:variant[][])  [unwired: 3 in, 1 out]
            n271 = xnode "Database Variant To Data"("database variant"=w983, "error in (no error)"=w977, "type"=string[][] [["", " "]]) -> ("data"=w982:string[][], "error out"=w976:errorcluster)
            n272 = property on="筛选结果" class="MCListbox (strict)"("ItemNames"=w982) -> ()  [unwired: 2 in, 2 out]
          }
        }
      }
    }
  }
  n273 = property on="筛选结果" class="MCListbox (strict)"("ItemNames"=w2) -> ()  [unwired: 2 in, 2 out]
  n274 = property on="预览数据" class="MCListbox (strict)"("ItemNames"=w2) -> ()  [unwired: 2 in, 2 out]
  n275 = invoke on="树形" class="Tree (严格)" method="Edit Tree Items.Delete"("Delete Children"=TRUE ("删除子项？")) -> ()  [unwired: 4 in, 5 out]
